vi "Set Cursor Unbusy.vi"(8 "error in (no error)":errorcluster, 11 "IViewManager In":refnum<class "IViewManager.lvclass">) -> (0 "error out":errorcluster, 3 "IViewManager Out":refnum<class "IViewManager.lvclass">)   [LabVIEW 2015, in "IViewManager.lvlib" / "IViewManager.lvclass"]
uses:
  IViewManager.lvclass
  IViewManager.lvclass/IViewManager.ctl
  <vilib>/ActorFramework/Message Enqueuer/Message Enqueuer.lvclass/Message Enqueuer.ctl
  <vilib>/ActorFramework/Message Enqueuer/Enqueue.vi
  <vilib>/ActorFramework/Message Priority Queue/Priority Enqueue.vi
  IViewable/IViewable/IViewable.lvclass
  IViewable/IViewable Messages/Set Cursor Unbusy Msg/Set Cursor Unbusy Msg.lvclass
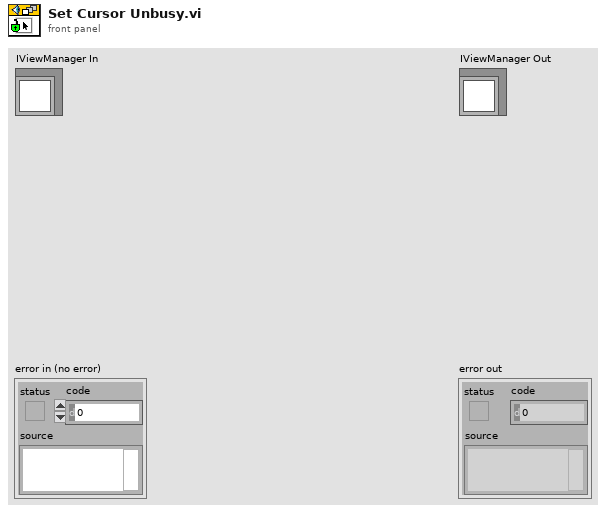
[diagram p1: front panel]
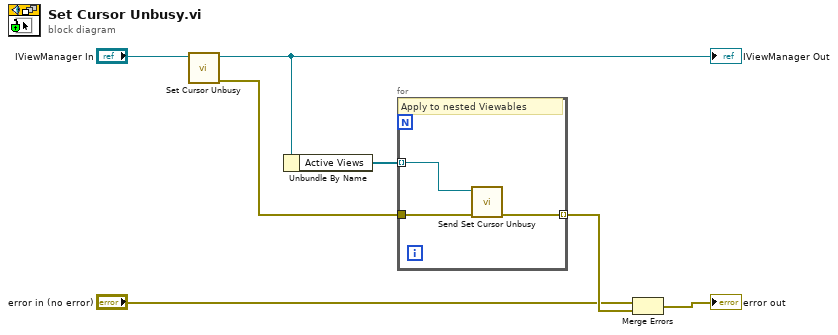
[diagram p0: block diagram]
diagram:
  n1 = call-parent "Set Cursor Unbusy.vi"("IViewable In"="IViewManager In") -> ("error out"=w7:errorcluster, "IViewable Out"=w2:refnum<class "IViewManager.lvclass">)  [unwired: 9 in]
  "IViewManager Out" <- w2
  n2 = Unbundle By Name(w2) -> ("Active Views"=w5:refnum<class "Message Enqueuer.lvclass">[])
  n3 = for {
    tunnel: w5 -> [w10] mode=indexing
    tunnel: w7 -> [w9]
    tunnel: [w8] -> w6 mode=indexing
    # "Apply to nested Viewables"
    n4 = call "Send Set Cursor Unbusy.vi"("error in (no error)"=w9, "Message Enqueuer"=w10) -> ("error out"=w8:errorcluster)  [unwired: 8 in, 1 out]
  }
  n5 = Merge Errors("error in (no error)", w6) -> (→"error out":errorcluster)
